vi "makeBinaryFile.vi"   [LabVIEW 2014]
types:
  T1 = enum16{"big-endian, network order", "native, host order", "little-endian"}
  T2 = enum16{"open", "replace", "create", "open or create", "replace or create", "replace or create with confirmation"}
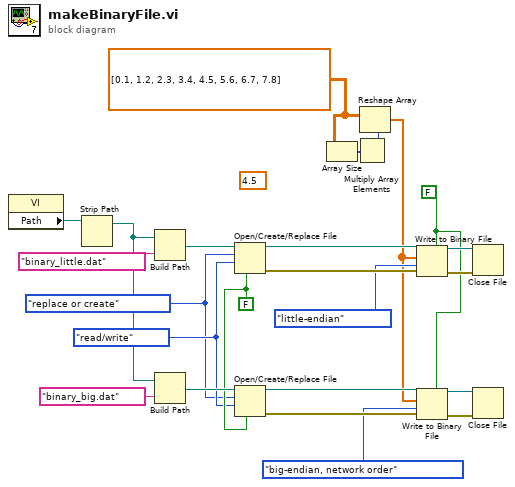
[diagram p0: block diagram]
diagram:
  (unwired) 4.5 ("Real Matrix Element")
  w10 = FALSE ("disable buffering (F)")
  w4 = dbl[][] [[0.1, 1.2, 2.3, 3.4], [4.5, 5.6, 6.7, 7.8]]
  w9 = FALSE ("prepend array or string size? (T)")
  w7 = enum16{"read/write", "read-only", "write-only"}."read/write" ("access (0:read/write)")
  w6 = T2."replace or create" ("operation (0:open)")
  n1 = property class="VI"() -> ("Path"=w24:path)  [unwired: 2 in, 2 out]
  n2 = Strip Path(path=w24) -> (stripped path=w5:path)  [unwired: 1 out]
  n3 = Build Path(base path=w5, name or relative path="binary_little.dat") -> (appended path=w23:path)
  n4 = Build Path(base path=w5, name or relative path="binary_big.dat") -> (appended path=w16:path)
  n5 = Open/Create/Replace File(file path (use dialog)=w23, operation (0:open)=w6, access (0:read/write)=w7, disable buffering (F)=w10) -> (refnum out=w21:refnum<file>, error out=w18:errorcluster)  [unwired: 2 in, 1 out]
  n6 = Open/Create/Replace File(file path (use dialog)=w16, operation (0:open)=w6, access (0:read/write)=w7, disable buffering (F)=w10) -> (refnum out=w14:refnum<file>, error out=w11:errorcluster)  [unwired: 2 in, 1 out]
  n7 = Array Size(array=w4) -> (size(s)=w3:i32[])
  n8 = Multiply Array Elements(1:w3) -> (0:w2:i32)
  n9 = Reshape Array(w4, w2) -> (w1:dbl[])
  n10 = Write to Binary File(file (use dialog)=w21, data=w1, error in=w18, 5:w9, 9:T1."little-endian" ("byte order (0:big-endian, network order)")) -> (refnum out=w19:refnum<file>, error out=w20:errorcluster)  [unwired: 1 in, 1 out]
  n11 = Write to Binary File(file (use dialog)=w14, data=w1, error in=w11, 5:w9, 9:T1."big-endian, network order" ("byte order (0:big-endian, network order)")) -> (refnum out=w12:refnum<file>, error out=w13:errorcluster)  [unwired: 1 in, 1 out]
  n12 = Close File(refnum=w19, error in=w20) -> ()  [unwired: 2 out]
  n13 = Close File(refnum=w12, error in=w13) -> ()  [unwired: 2 out]
